vi "PXI-DAQ Status.vi"(11 "error in (no error)":errorcluster) -> (8 "Finished?":bool, 15 "error out":errorcluster)   [LabVIEW 2020]
uses:
  DAQ Engine VIs/PXI Globals.vi
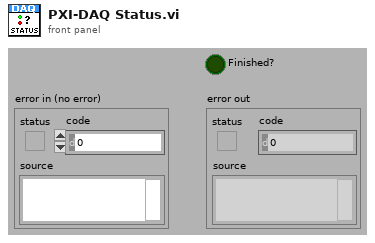
[diagram p1: front panel]
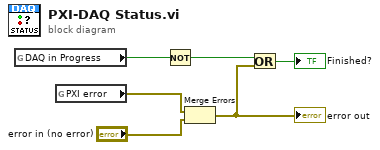
[diagram p0: block diagram]
diagram:
  n1 = global read "PXI Globals.vi" "DAQ in Progress"() -> (w4:bool)
  n2 = global read "PXI Globals.vi" "PXI error"() -> (w6:errorcluster)
  n3 = Not(x=w4) -> (.not. x?=w2:bool)
  n4 = Merge Errors(w6, "error in (no error)") -> (w1:errorcluster)
  "error out" <- w1
  n5 = Or(x=w2, y=w1) -> (x .or. y?=→"Finished?":bool)
